vi "Get Move Group Along A Line Status.vi"(4 "error in (no error)":errorcluster, 6 "Group Number (1)":i32=1 min=1, 7 "VISA resource name":refnum<visa-resource-name>) -> (0 "error out":errorcluster, 2 "Positons (units)":dbl[](array[numeric]), 3 "VISA resource name out":refnum<visa-resource-name>)   [LabVIEW 2018, in "Newport ESP301.lvlib"]
doc: "Get the target positions of axes assigned to the group."
uses:
  Newport ESP301.lvlib
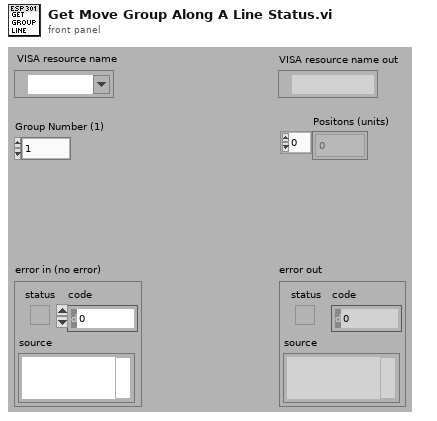
[diagram p1: front panel]
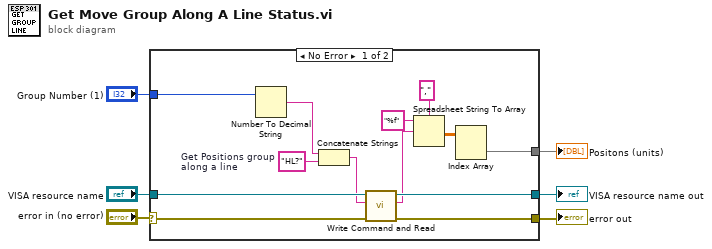
[diagram p0: block diagram]
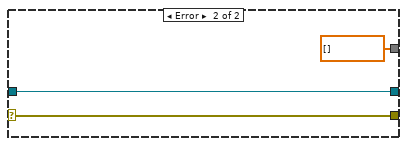
[diagram p2: hidden frame]
diagram:
  n1 = case shown="No Error" "error in (no error)" {
    selector: "error in (no error)" -> [w16 w22]
    tunnel: [w18 w22] -> w6
    tunnel: "VISA resource name" -> [w19 w21]
    tunnel: [w17 w21] -> w5
    tunnel: "Group Number (1)" -> [w12 _]
    tunnel: [w7 dbl[] []] -> w1
    frame No Error {
      w15 = "HL?"  # Get Positions group  along a line
      n2 = Number To Decimal String(number=w12) -> (decimal integer string=w14:string)  [unwired: 1 in]
      n3 = Concatenate Strings(w14, w15) -> (w13:string)
      n4 = call "Write Command and Read.vi"("error in (no error)"=w16, "Command"=w13, "VISA resource name"=w19) -> ("error out"=w18:errorcluster, "Returned string"=w10:string, "VISA resource name out"=w17:refnum<visa-resource-name>)  [unwired: 4 in]
      n5 = Spreadsheet String To Array(delimiter (Tab)="," ("séparateur (Tabulation)"), format string="%f" ("chaîne de format"), spreadsheet string=w10) -> (array=w9:dbl[][])  [unwired: 1 in]
      n6 = Index Array(array=w9) -> (element=w7:dbl[])  [unwired: 2 in]
    }
    frame Error {
    }
  }
  "error out" <- w6
  "VISA resource name out" <- w5
  "Positons (units)" <- w1
